vi "Create Spectra Figure.vi"() -> ()   [LabVIEW 2020]
uses:
  <vilib>/Heliosphere Research LLC/Advanced Plotting Toolkit/api_core/NewPlotProperties.ctl
  <vilib>/Heliosphere Research LLC/Advanced Plotting Toolkit/typedefs/PlotColor.ctl
  <vilib>/Heliosphere Research LLC/Advanced Plotting Toolkit/api_annotations/LabelProperties.ctl
  <vilib>/Heliosphere Research LLC/Advanced Plotting Toolkit/properties/Text.ctl
  <vilib>/Heliosphere Research LLC/Advanced Plotting Toolkit/properties/Text_FontSize.ctl
  <vilib>/Heliosphere Research LLC/Advanced Plotting Toolkit/properties/Text_FontStyle.ctl
  <vilib>/Heliosphere Research LLC/Advanced Plotting Toolkit/api_figure/TicksProperties.ctl
  <vilib>/Heliosphere Research LLC/Advanced Plotting Toolkit/api_plotting/LineProperties.ctl
  <vilib>/Heliosphere Research LLC/Advanced Plotting Toolkit/properties/Line.ctl
  <vilib>/Heliosphere Research LLC/Advanced Plotting Toolkit/properties/Line_Style.ctl
  <vilib>/Heliosphere Research LLC/Advanced Plotting Toolkit/properties/Marker.ctl
  <vilib>/Heliosphere Research LLC/Advanced Plotting Toolkit/properties/Marker_Style.ctl
  <vilib>/Heliosphere Research LLC/Advanced Plotting Toolkit/properties/Display.ctl
  <vilib>/regexp/Match Regular Expression.xnode
  <vilib>/Heliosphere Research LLC/Advanced Plotting Toolkit/Advanced Plotting Toolkit.lvlib
  <vilib>/Analysis/NI_AALPro.lvlib
panel:
  out "Bar Plot":picture
  out "Pressure":picture
  out "Speed Profiles":picture
  out "Full Spectrum":picture
  out "Trimmed Spectra":picture
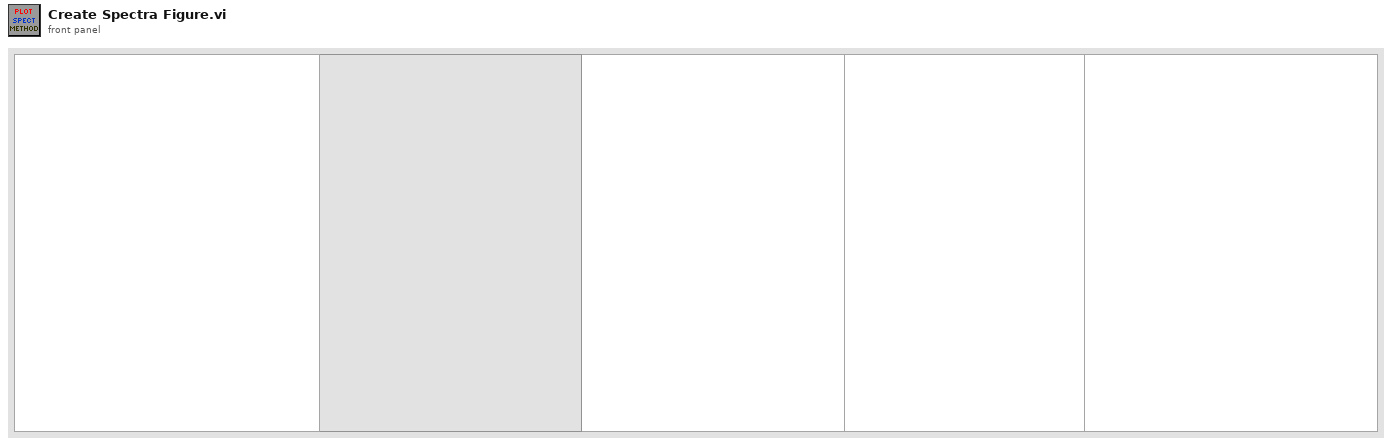
[diagram p1: front panel]
types:
  T1 = typedef "Advanced Plotting Toolkit.lvlib/LabelProperties.ctl" = cluster{"Text":T2}
  T2 = typedef "Advanced Plotting Toolkit.lvlib/Text.ctl" = cluster{"Color":T3, "Background Color":T3, "Font Size (points)":T4, "Font Style":T5, "Rotation Angle":dbl}
  T3 = typedef "Advanced Plotting Toolkit.lvlib/PlotColor.ctl" = u32
  T4 = typedef "Advanced Plotting Toolkit.lvlib/Text_FontSize.ctl" = i32
  T5 = typedef "Advanced Plotting Toolkit.lvlib/Text_FontStyle.ctl" = enum16{"Automatic", "Normal", "Italic", "Bold"}
  T6 = typedef "Advanced Plotting Toolkit.lvlib/TicksProperties.ctl" = cluster{"Text":T2}
  T7 = typedef "Advanced Plotting Toolkit.lvlib/NewPlotProperties.ctl" = cluster{"Background Color":T3, "Axis Background":T3, "Left Margin":dbl, "Right Margin":dbl, "Bottom Margin":dbl, "Top Margin":dbl, "Aspect Ratio":dbl}
  T8 = typedef "Advanced Plotting Toolkit.lvlib/PlotID.ctl" = i32
  T9 = typedef "Advanced Plotting Toolkit.lvlib/LineProperties.ctl" = cluster{"Line":T10, "Marker":T12, "Display":T14}
  T10 = typedef "Advanced Plotting Toolkit.lvlib/Line.ctl" = cluster{"Style":T11, "Color":T3, "Width":sgl}
  T11 = typedef "Advanced Plotting Toolkit.lvlib/Line_Style.ctl" = enum16{"Automatic", "Solid", "Dashed", "Dotted", "Dash-dot", "Invisible"}
  T12 = typedef "Advanced Plotting Toolkit.lvlib/Marker.ctl" = cluster{"Style":T13, "Color":T3, "Size":dbl}
  T13 = typedef "Advanced Plotting Toolkit.lvlib/Marker_Style.ctl" = enum16{"Automatic", "Circle", "Square", "Triangle", "Diamond", "Star", "Invisible"}
  T14 = typedef "Advanced Plotting Toolkit.lvlib/Display.ctl" = cluster{"Alpha":dbl, "Z Order":dbl}
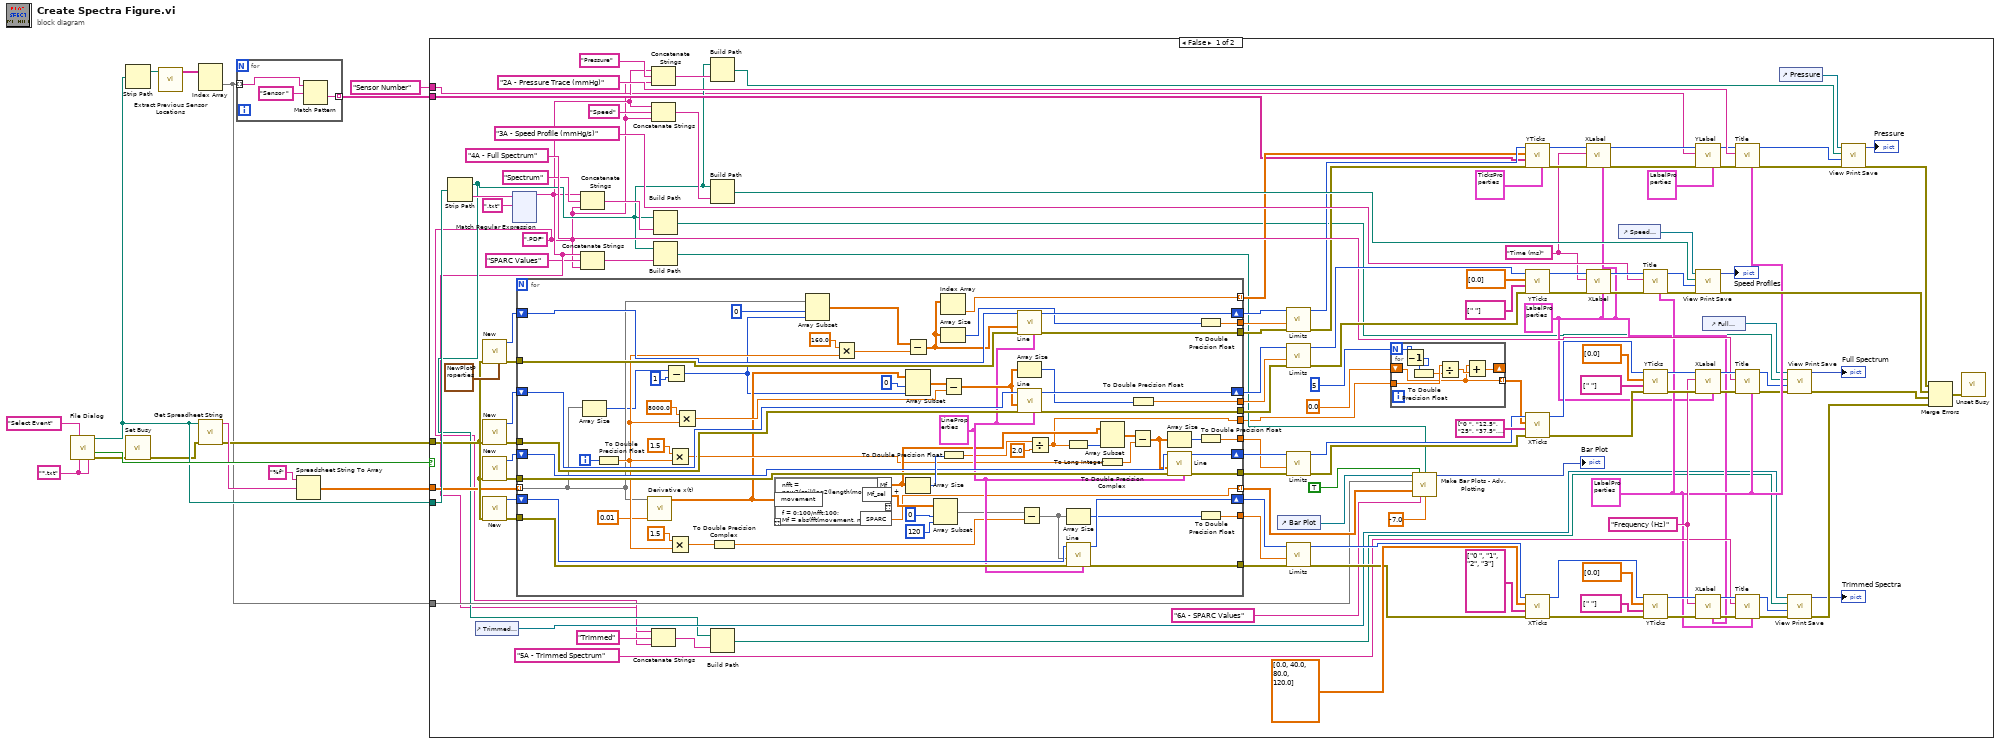
[diagram p0: block diagram]
diagram:
  w12 = "*.txt" ("pattern label")
  n1 = call "File Dialog"("prompt"="Select Event", "pattern (all files)"=w12, "pattern label"=w12) -> ("selected path"=w5:path, "cancelled"=w14:bool, "error out"=w4:errorcluster)  [unwired: 9 in, 1 out]
  n2 = Strip Path(path=w5) -> (stripped path=w10:path)  [unwired: 1 out]
  n3 = call <vilib>:"Set Busy.vi"("error in (no error)"=w4) -> ("error out"=w3:errorcluster)  [unwired: 9 in, 1 out]
  n4 = call "Extract Previous Sensor Locations.vi"("Folder Path"=w10) -> ("Sensors"=w9:string[][])  [unwired: 8 in, 2 out]
  n5 = Index Array(array=w9) -> (element=w2:string[])  [unwired: 2 in]
  n6 = call "Get Spreadheet String.vi"("error in (no error)"=w3, "File Path"=w5) -> ("error out"=w6:errorcluster, "Spreadsheet String"=w7:string)  [unwired: 8 in]
  n7 = for {
    tunnel: w2 -> [w18] mode=indexing
    tunnel: [w16] -> w8 mode=indexing
    n8 = Match Pattern(string=w18, regular expression="Sensor ") -> (after substring=w16:string)  [unwired: 1 in, 3 out]
  }
  n9 = Spreadsheet String To Array(format string="%f", spreadsheet string=w7) -> (array=w11:dbl[][])  [unwired: 2 in]
  n10 = case shown="False" w14 {
    tunnel: w6 -> [w82 _]
    tunnel: w11 -> [w65 _]
    tunnel: w5 -> [w92 _]
    tunnel: w8 -> [w49 _]
    tunnel: w2 -> [w47 _]
    tunnel: "Sensor Number" ("Label") -> [w34 _]
    frame False {
      w32 = ".PDF" ("string")
      w74 = T1 {"Text"={"Color"=2147483647, "Background Color"=2147483647, "Font Size (points)"=-4, "Font Style"=enum."Bold", "Rotation Angle"=nan}} ("Properties")
      w73 = T1 {"Text"={"Color"=2147483647, "Background Color"=2147483647, "Font Size (points)"=-3, "Font Style"=enum."Bold", "Rotation Angle"=nan}} ("Properties")
      w102 = "Frequency (Hz)" ("Label")
      w68 = "Time (ms)" ("Label")
      n11 = Strip Path(path=w92) -> (stripped path=w43:path, name=w91:string)
      n12 = control-ref of="Trimmed Spectra"() -> (w55:refnum<vi>)
      n13 = call <vilib>:"New.vi"("Properties"=T7 {"Background Color"=2147483647, "Axis Background"=2147483647, "Left Margin"=0.15, "Right Margin"=nan, "Bottom Margin"=nan, "Top Margin"=nan, "Aspect Ratio"=nan}, "error in (no error)"=w82) -> ("error out"=w146:errorcluster, "Plot ID"=w145:T8)  [unwired: 8 in]
      n14 = call <vilib>:"New.vi"("error in (no error)"=w82) -> ("error out"=w140:errorcluster, "Plot ID"=w143:T8)  [unwired: 9 in]
      n15 = call <vilib>:"New.vi"("error in (no error)"=w82) -> ("error out"=w139:errorcluster, "Plot ID"=w144:T8)  [unwired: 9 in]
      n16 = call <vilib>:"New.vi"("error in (no error)"=w82) -> ("error out"=w138:errorcluster, "Plot ID"=w142:T8)  [unwired: 9 in]
      n17 = xnode "Match Regular Expression"("input string"=w91, "regular expression"=".txt") -> ("before match"=w41:string)  [unwired: 4 in, 4 out]
      n18 = for {
        tunnel: w146 -> [w328]
        tunnel: [w325] -> w69
        shift-right: [w326] -> w70
        shift-left: w145 -> [w327]
        shift-right: [w319] -> w124
        shift-left: w143 -> [w324]
        shift-right: [w320] -> w118
        shift-left: w144 -> [w323]
        shift-right: [w321] -> w116
        shift-left: w142 -> [w322]
        tunnel: w140 -> [w318]
        tunnel: w139 -> [w317]
        tunnel: w138 -> [w316]
        tunnel: [w315] -> w123
        tunnel: [w314] -> w119
        tunnel: [w313] -> w115
        tunnel: [w302] -> w71
        tunnel: [w299] -> w122
        tunnel: [w294] -> w117
        tunnel: [w293] -> w114
        tunnel: [w271] -> w75 mode=indexing
        tunnel: w65 -> [w276] mode=indexing
        tunnel: [w270] -> w48 mode=indexing
        tunnel: [w268] -> w37
        i -> [w312]
        w288 = T9 {"Line"={"Style"=enum."Automatic", "Color"=2147483647, "Width"=2.0}, "Marker"={"Style"=enum."Automatic", "Color"=2147483647, "Size"=nan}, "Display"={"Alpha"=nan, "Z Order"=nan}} ("Properties")
        n19 = Array Size(array=w276) -> (size(s)=w275:i32)
        n20 = To Double Precision Float(number=w312) -> (double precision float=w308:dbl)
        n21 = call <vilib>:"Derivative x(t).vi"("dt"=0.01, "X"=w276) -> ("dX/dt"=w279:dbl[])  [unwired: 8 in, 1 out]
        n22 = Subtract(x=w275, y=1) -> (x-y=w273:i32)
        n23 = Multiply(x=1.5, y=w308) -> (x*y=w283:dbl)
        n24 = Multiply(x=1.5, y=w308) -> (x*y=w280:dbl)
        n25 = Multiply(x=8000.0, y=w308) -> (x*y=w307:dbl)
        n26 = To Double Precision Complex(1:w280) -> (0:w281:cdb)
        n27 = script code="nfft = pow2(ceil(log2(length(movement))) + 4);\n\nf = 0:100/nfft:100;\nMf = abs(fft(movement, nfft));\nMf = Mf/max(Mf);\n\nfc_inx = find(f<=3);\nf_sel = f(fc_inx);\nMf_sel = Mf(fc_inx);\n\n\ninx = find((Mf_sel>=0.01));\nfc_inx = inx(1):inx(end);\nf_sel = f_sel(fc_inx);\nMf_sel = Mf_sel(fc_inx);\n\nSPARC = -sum(sqrt((diff(f_sel)/f_sel(end)-f_sel(1)).^2+(diff(Mf_sel).^2)));"("movement"=w279) -> ("Mf"=w284:cdb[], "Mf_sel"=w285:cdb[], "SPARC"=w270:dbl)  [unwired: 1 in, 1 out]
        n28 = Array Subset(array=w276, index=0, length=w273) -> (w278:dbl[])
        n29 = Multiply(x=160.0, y=w308) -> (x*y=w309:dbl)
        n30 = Subtract(x=w278, y=w309) -> (x-y=w272:dbl[])
        n31 = Array Subset(array=w279, index=0, length=w273) -> (w277:dbl[])
        n32 = Array Size(array=w284) -> (size(s)=w331:i32)
        n33 = Array Subset(array=w285, index=0, length=120) -> (w287:cdb[])
        n34 = Index Array(array=w272) -> (element=w271:dbl)  [unwired: 1 in]
        n35 = Array Size(array=w272) -> (size(s)=w303:i32)
        n36 = Subtract(x=w277, y=w307) -> (x-y=w300:dbl[])
        n37 = To Double Precision Float(number=w331) -> (double precision float=w269:dbl)
        n38 = call <vilib>:"Line.vi"("Properties"=w288, "error in (no error)"=w328, "Y Data"=w272, "Plot ID"=w327) -> ("error out"=w325:errorcluster, "Plot ID out"=w326:T8)  [unwired: 6 in]
        n39 = Array Size(array=w300) -> (size(s)=w301:i32)
        n40 = call <vilib>:"Line.vi"("Properties"=w288, "error in (no error)"=w318, "Y Data"=w300, "Plot ID"=w324) -> ("error out"=w315:errorcluster, "Plot ID out"=w319:T8)  [unwired: 6 in]
        n41 = Subtract(x=w287, y=w281) -> (x-y=w295:cdb[])
        n42 = Divide(x=w269, y=2.0) -> (x/y=w268:dbl)
        n43 = To Long Integer(number=w268) -> (32bit integer=w329:i32)
        n44 = Array Size(array=w295) -> (size(s)=w296:i32)
        n45 = call <vilib>:"Line.vi"("Properties"=w288, "error in (no error)"=w316, "Y Data"=w295, "Plot ID"=w322) -> ("error out"=w313:errorcluster, "Plot ID out"=w321:T8)  [unwired: 6 in]
        n46 = Array Subset(array=w284, length=w329) -> (w311:cdb[])  [unwired: 1 in]
        n47 = To Double Precision Complex(1:w283) -> (0:w282:cdb)
        n48 = Subtract(x=w311, y=w282) -> (x-y=w297:cdb[])
        n49 = To Double Precision Float(number=w301) -> (double precision float=w299:dbl)
        n50 = Array Size(array=w297) -> (size(s)=w298:i32)
        n51 = call <vilib>:"Line.vi"("Properties"=w288, "error in (no error)"=w317, "Y Data"=w297, "Plot ID"=w323) -> ("error out"=w314:errorcluster, "Plot ID out"=w320:T8)  [unwired: 6 in]
        n52 = To Double Precision Float(number=w303) -> (double precision float=w302:dbl)
        n53 = To Double Precision Float(number=w298) -> (double precision float=w294:dbl)
        n54 = To Double Precision Float(number=w296) -> (double precision float=w293:dbl)
      }
      n55 = Concatenate Strings(w41, "Spectrum" ("string"), w32) -> (w85:string)
      n56 = Concatenate Strings(w41, "SPARC Values" ("string"), w32) -> (w42:string)
      n57 = Concatenate Strings(w41, "Pressure" ("string"), w32) -> (w80:string)
      n58 = Concatenate Strings(w41, "Speed" ("string"), w32) -> (w88:string)
      n59 = Concatenate Strings(w41, "Trimmed" ("string"), w32) -> (w83:string)
      n60 = Build Path(base path=w43, name or relative path=w85) -> (appended path=w57:path)
      n61 = Build Path(base path=w43, name or relative path=w42) -> (appended path=w44:path)
      n62 = Build Path(base path=w43, name or relative path=w80) -> (appended path=w51:path)
      n63 = Build Path(base path=w43, name or relative path=w88) -> (appended path=w87:path)
      n64 = Build Path(base path=w43, name or relative path=w83) -> (appended path=w54:path)
      n65 = control-ref of="Bar Plot"() -> (w50:refnum<vi>)
      n66 = call <vilib>:"Limits.vi"("error in (no error)"=w69, "X Max"=w71, "Plot ID"=w70) -> ("error out"=w79:errorcluster, "Plot ID Out"=w78:T8)  [unwired: 7 in]
      n67 = call <vilib>:"Limits.vi"("error in (no error)"=w123, "X Max"=w122, "Plot ID"=w124) -> ("error out"=w103:errorcluster, "Plot ID Out"=w104:T8)  [unwired: 7 in]
      n68 = call <vilib>:"Limits.vi"("error in (no error)"=w119, "X Max"=w117, "Plot ID"=w118) -> ("error out"=w120:errorcluster, "Plot ID Out"=w121:T8)  [unwired: 7 in]
      n69 = call <vilib>:"Limits.vi"("error in (no error)"=w115, "X Max"=w114, "Plot ID"=w116) -> ("error out"=w112:errorcluster, "Plot ID Out"=w113:T8)  [unwired: 7 in]
      n70 = for {
        N: 5 -> [w147]
        shift-right: [w149] -> _
        shift-left: 0.0 -> [w150]
        tunnel: w37 -> [w153]
        tunnel: [w150] -> w36 mode=indexing
        n71 = Decrement(x=w147) -> (x-1=w148:i32)
        n72 = To Double Precision Float(number=w148) -> (double precision float=w152:dbl)
        n73 = Divide(x=w153, y=w152) -> (x/y=w151:dbl)
        n74 = Add(x=w150, y=w151) -> (x+y=w149:dbl)
      }
      n75 = call "Make Bar Plots - Adv. Plotting.vi"("Picture in"=w50, "Save Plot?"=TRUE, "Save Path"=w44, "Labels"=w47, "SPARC"=w48, "Title"="6A - SPARC Values", "Y Min"=-7.0) -> ("Picture"=→"Bar Plot":picture)  [unwired: 7 in, 1 out]
      n76 = call <vilib>:"YTicks.vi"("Properties"=T6 {"Text"={"Color"=2147483647, "Background Color"=2147483647, "Font Size (points)"=-3, "Font Style"=enum."Bold", "Rotation Angle"=0.0}} ("Senor Label Props"), "error in (no error)"=w79, "Tick Labels"=w49, "Tick Locations"=w75, "Plot ID"=w78) -> ("error out"=w76:errorcluster, "Plot ID Out"=w77:T8)  [unwired: 5 in]
      n77 = call <vilib>:"YTicks.vi"("error in (no error)"=w103, "Tick Labels"=string[] [" "], "Tick Locations"=dbl[] [0.0], "Plot ID"=w104) -> ("error out"=w108:errorcluster, "Plot ID Out"=w107:T8)  [unwired: 6 in]
      n78 = call <vilib>:"XTicks.vi"("error in (no error)"=w120, "Tick Labels"=string[] ["0 ", "12.5", "25", "37.5", "50"], "Tick Locations"=w36, "Plot ID"=w121) -> ("error out"=w129:errorcluster, "Plot ID Out"=w125:T8)  [unwired: 6 in]
      n79 = call <vilib>:"XTicks.vi"("error in (no error)"=w112, "Tick Labels"=string[] ["0 ", "1", "2", "3"], "Tick Locations"=dbl[] [0.0, 40.0, 80.0, 120.0], "Plot ID"=w113) -> ("error out"=w134:errorcluster, "Plot ID Out"=w130:T8)  [unwired: 6 in]
      n80 = call <vilib>:"XLabel.vi"("Properties"=w73, "error in (no error)"=w76, "Label"=w68, "Plot ID"=w77) -> ("error out"=w63:errorcluster, "Plot ID out"=w64:T8)  [unwired: 6 in]
      n81 = call <vilib>:"XLabel.vi"("Properties"=w73, "error in (no error)"=w108, "Label"=w68, "Plot ID"=w107) -> ("error out"=w95:errorcluster, "Plot ID out"=w96:T8)  [unwired: 6 in]
      n82 = control-ref of="Speed Profiles"() -> (w141:refnum<vi>)
      n83 = call <vilib>:"Title.vi"("Properties"=w74, "error in (no error)"=w95, "Title"="3A - Speed Profile (mmHg/s)", "Plot ID"=w96) -> ("error out"=w26:errorcluster, "Plot ID out"=w25:T8)  [unwired: 6 in]
      n84 = call <vilib>:"YTicks.vi"("error in (no error)"=w129, "Tick Labels"=string[] [" "], "Tick Locations"=dbl[] [0.0], "Plot ID"=w125) -> ("error out"=w109:errorcluster, "Plot ID Out"=w106:T8)  [unwired: 6 in]
      n85 = call <vilib>:"YTicks.vi"("error in (no error)"=w134, "Tick Labels"=string[] [" "], "Tick Locations"=dbl[] [0.0], "Plot ID"=w130) -> ("error out"=w110:errorcluster, "Plot ID Out"=w105:T8)  [unwired: 6 in]
      n86 = call <vilib>:"YLabel.vi"("Properties"=T1 {"Text"={"Color"=2147483647, "Background Color"=2147483647, "Font Size (points)"=-3, "Font Style"=enum."Bold", "Rotation Angle"=nan}}, "error in (no error)"=w63, "Label"=w34, "Plot ID"=w64) -> ("error out"=w61:errorcluster, "Plot ID out"=w62:T8)  [unwired: 6 in]
      n87 = call "View Print Save.vi"("error in (no error)"=w26, "Plot ID in"=w25, "appended path"=w87, "Picture in"=w141) -> ("error out"=w137:errorcluster, "Picture"=→"Speed Profiles":picture)  [unwired: 6 in]
      n88 = call <vilib>:"XLabel.vi"("Properties"=w73, "error in (no error)"=w109, "Label"=w102, "Plot ID"=w106) -> ("error out"=w98:errorcluster, "Plot ID out"=w97:T8)  [unwired: 6 in]
      n89 = call <vilib>:"XLabel.vi"("Properties"=w73, "error in (no error)"=w110, "Label"=w102, "Plot ID"=w105) -> ("error out"=w101:errorcluster, "Plot ID out"=w100:T8)  [unwired: 6 in]
      n90 = control-ref of="Full Spectrum"() -> (w58:refnum<vi>)
      n91 = call <vilib>:"Title.vi"("Properties"=w74, "error in (no error)"=w61, "Title"="2A - Pressure Trace (mmHg)", "Plot ID"=w62) -> ("error out"=w20:errorcluster, "Plot ID out"=w19:T8)  [unwired: 6 in]
      n92 = call <vilib>:"Title.vi"("Properties"=w74, "error in (no error)"=w98, "Title"="4A - Full Spectrum", "Plot ID"=w97) -> ("error out"=w22:errorcluster, "Plot ID out"=w21:T8)  [unwired: 6 in]
      n93 = call <vilib>:"Title.vi"("Properties"=w74, "error in (no error)"=w101, "Title"="5A - Trimmed Spectrum", "Plot ID"=w100) -> ("error out"=w23:errorcluster, "Plot ID out"=w24:T8)  [unwired: 6 in]
      n94 = control-ref of="Pressure"() -> (w52:refnum<vi>)
      n95 = call "View Print Save.vi"("error in (no error)"=w22, "Plot ID in"=w21, "appended path"=w57, "Picture in"=w58) -> ("error out"=w59:errorcluster, "Picture"=→"Full Spectrum":picture)  [unwired: 6 in]
      n96 = call "View Print Save.vi"("error in (no error)"=w23, "Plot ID in"=w24, "appended path"=w54, "Picture in"=w55) -> ("error out"=w56:errorcluster, "Picture"=→"Trimmed Spectra":picture)  [unwired: 6 in]
      n97 = call "View Print Save.vi"("error in (no error)"=w20, "Plot ID in"=w19, "appended path"=w51, "Picture in"=w52) -> ("error out"=w53:errorcluster, "Picture"=→"Pressure":picture)  [unwired: 6 in]
      n98 = Merge Errors(w53, w137, w59, w56) -> (w35:errorcluster)
      n99 = call <vilib>:"Unset Busy.vi"("error in (no error)"=w35) -> ()  [unwired: 10 in, 1 out]
    }
    frame True {
    }
  }
